vi "Operation(SubVI).vi"(1 "OPERATION":T1) -> ()   [LabVIEW 2018]
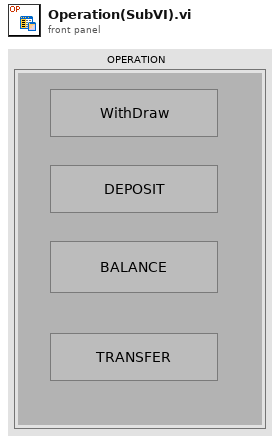
[diagram p1: front panel]
types:
  T1 = cluster{"WITHDRAW":bool, "DEPOSIT":bool, "BALANCE ":bool, "TRANSFER":bool}
  T2 = enum16{"LOGIN", "OPERATION", "WITHDRAW", "DEPOSIT", "BALANCE", "TRANSFER"}
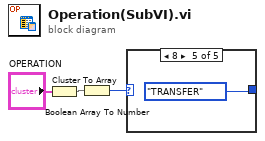
[diagram p0: block diagram]
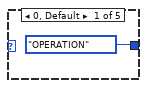
[diagram p2: hidden frame]
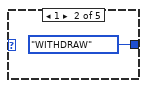
[diagram p3: hidden frame]
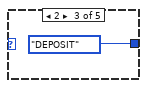
[diagram p4: hidden frame]
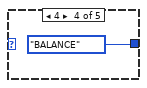
[diagram p5: hidden frame]
diagram:
  n1 = Cluster To Array(cluster="OPERATION") -> (array=w3:bool[])
  n2 = Boolean Array To Number(Boolean array=w3) -> (number=w1:u32)
  n3 = case shown="8" w1 {
    tunnel: [T2."OPERATION" T2."WITHDRAW" T2."DEPOSIT" T2."BALANCE" T2."TRANSFER"] -> _
    frame 0, Default {
    }
    frame 1 {
    }
    frame 2 {
    }
    frame 4 {
    }
    frame 8 {
    }
  }
